vi "Read Error Handling Parameters.vi"(4 "Error In":errorcluster, 7 "DB_ADO in":refnum<class "Config Data_DB_ADO.lvclass">) -> (0 "Error Out":errorcluster, 1 "Buttons":T1={"Continue/Ok Button"="Continue", "Stop Button"="Stop"}, 2 "Action":T2(ring), 3 "DB_ADO out":refnum<class "Config Data_DB_ADO.lvclass">)   [LabVIEW 2015, in "Config Data.lvlib" / "Config Data_DB_ADO.lvclass"]
uses:
  Config Data_DB_ADO.lvclass
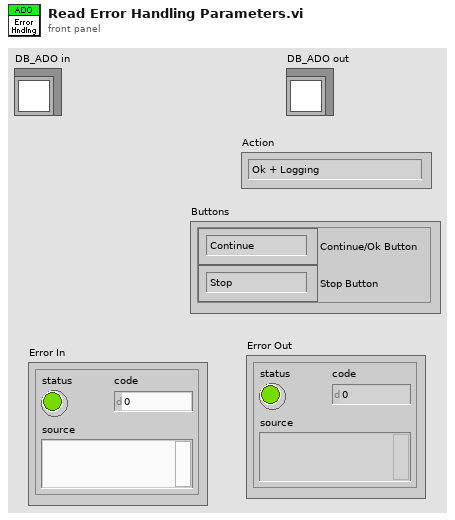
[diagram p1: front panel]
types:
  T1 = cluster{"Continue/Ok Button":string, "Stop Button":string}
  T2 = enum16{"Ok + Logging", "Continue/Stop + Logging", "Logging Only", "Ok Only", "Continue/Stop Only"}
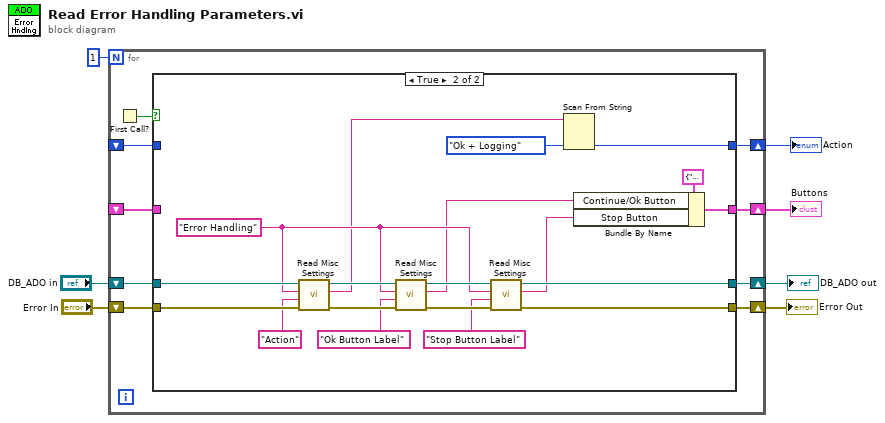
[diagram p0: block diagram]
diagram:
  n1 = for {
    N: 1 -> [_]
    shift-right: [w13] -> w4
    shift-left: "DB_ADO in" -> [w16]
    shift-right: [w14] -> w5
    shift-left: "Error In" -> [w15]
    shift-right: [w12] -> w3
    shift-left: _ -> [w10]
    shift-right: [w11] -> w2
    shift-left: _ -> [w8]
    n2 = First Call?() -> (First Call?: T/F=w9:bool)
    n3 = case shown="True" w9 {
      tunnel: w16 -> [w20 w39]
      tunnel: w15 -> [w19 w38]
      tunnel: [w19 w35] -> w14
      tunnel: [w20 w32] -> w13
      tunnel: [w18 w28] -> w12
      tunnel: [w17 w24] -> w11
      tunnel: w10 -> [w18 _]
      tunnel: w8 -> [w17 _]
      frame False {
      }
      frame True {
        w31 = "Error Handling" ("Section")
        n4 = call-dynamic "Read Misc Settings.vi"("error in (no error)"=w38, "Key"="Action" ("default value"), "Section"=w31, "DB_ADO in"=w39) -> ("error out"=w37:errorcluster, "p_value"=w29:string, "DB_ADO out"=w33:refnum<class "Config Data_DB_ADO.lvclass">)  [unwired: 2 in]
        n5 = call-dynamic "Read Misc Settings.vi"("error in (no error)"=w37, "Key"="Ok Button Label" ("default value"), "Section"=w31, "DB_ADO in"=w33) -> ("error out"=w36:errorcluster, "p_value"=w26:string, "DB_ADO out"=w34:refnum<class "Config Data_DB_ADO.lvclass">)  [unwired: 2 in]
        n6 = call-dynamic "Read Misc Settings.vi"("error in (no error)"=w36, "Key"="Stop Button Label" ("default value"), "Section"=w31, "DB_ADO in"=w34) -> ("error out"=w35:errorcluster, "p_value"=w25:string, "DB_ADO out"=w32:refnum<class "Config Data_DB_ADO.lvclass">)  [unwired: 2 in]
        n7 = Scan From String(input string=w29, default 1=T2."Ok + Logging" ("Action")) -> (output 1=w28:T2)  [unwired: 3 in, 3 out]
        n8 = Bundle By Name(cluster=T1 {"Continue/Ok Button"="Continue", "Stop Button"="Stop"} ("Buttons"), "Continue/Ok Button"=w26, "Stop Button"=w25) -> (w24:T1)
      }
    }
  }
  "Error Out" <- w5
  "DB_ADO out" <- w4
  "Buttons" <- w2
  "Action" <- w3
